vi "LINC Add Packet.vi"(0 "LINC session":refnum<class "LINC.lvclass">, 1 "add header (F)":bool, 2 "type (CMD)":enum16{"CMD", "TLM"}(ring), 5 "item names in":string[](array[string]), 7 "item formats in":T1[](array[typedef]), 9 "hazardous":bool, 11 "e rror in (no error)":errorcluster, 12 "packet name":string, 13 "packet description":string, 14 "ID":i32) -> (4 "dup LINC session":refnum<class "LINC.lvclass">, 15 "error out":errorcluster)   [LabVIEW 2018, in "STEPkgDriver_LINC.lvlib" / "LINC.lvclass"]
uses:
  LINC.lvclass
  STEPkgDriver_LINC.lvlib
  LINC Global Mode.ctl
  LINC Global ID Mode.ctl
  LINC Format Prototype.ctl
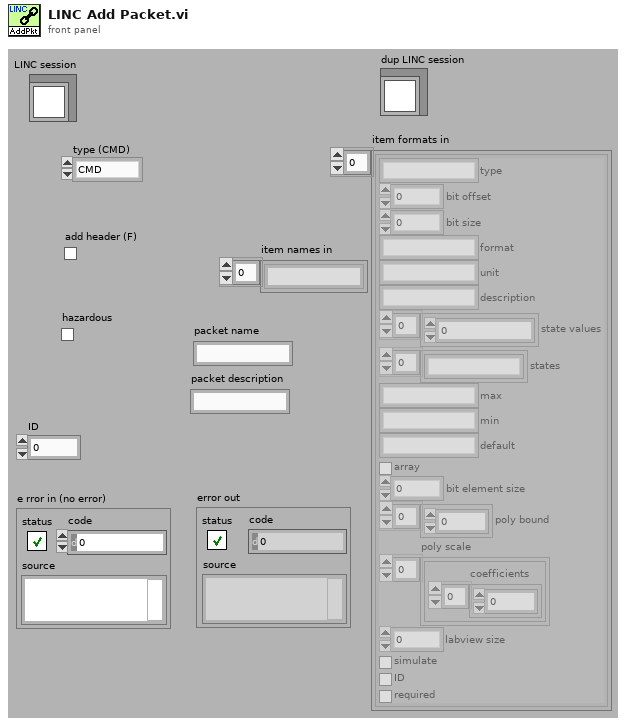
[diagram p1: front panel]
types:
  T1 = typedef "STEPkgDriver_LINC.lvlib/LINC Format Prototype.ctl" = cluster{"type":string, "bit offset":i32, "bit size":i32, "format":string, "unit":string, "description":string, "state values":i64[], "states":string[], "max":string, "min":string, "default":string, "array":bool, "bit element size":i32, "poly bound":dbl[], "poly scale":cluster{"coefficients":dbl[]}[], "labview size":i32, "simulate":bool, "ID":bool, "required":bool}
  T2 = typedef "STEPkgDriver_LINC.lvlib/LINC Global ID Mode.ctl" = enum16{"INIT", "CLEAR", "GET_ID"}
  T3 = typedef "STEPkgDriver_LINC.lvlib/LINC Global Mode.ctl" = enum16{"INIT", "CLEAR", "ADD_PKT_HDR", "ADD_PKT", "GET_PKT_NAMES", "GET_PKT_DESC", "GET_PKT_HDR", "GET_PKT", "SET_PKT", "SET_DATA", "SIM_EN", "SIM_DS"}
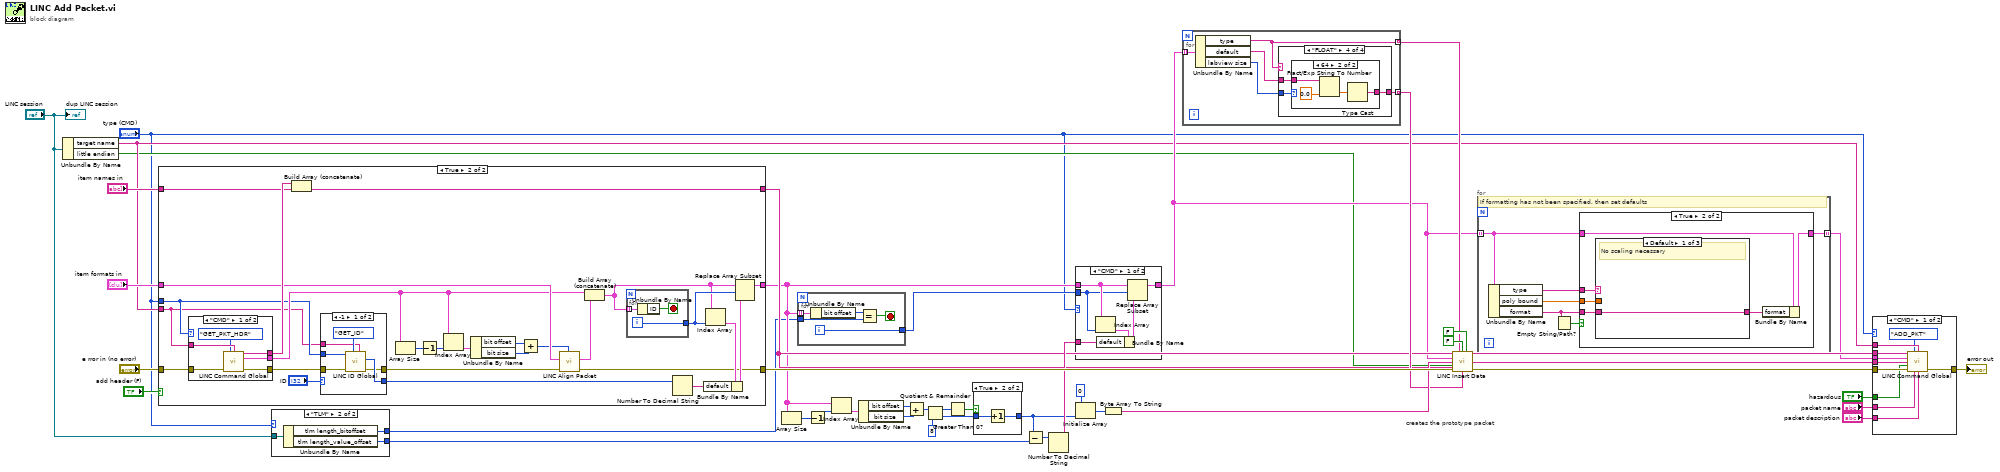
[diagram p0: block diagram]
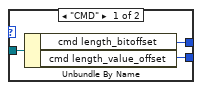
[diagram p4: hidden frame]
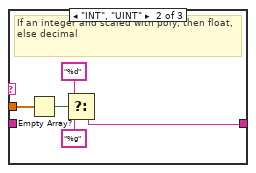
[diagram p6: hidden frame]
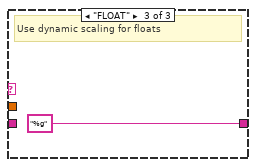
[diagram p7: hidden frame]
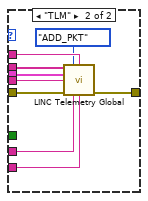
[diagram p8: hidden frame]
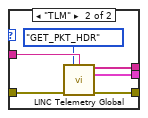
[diagram p11: hidden frame]
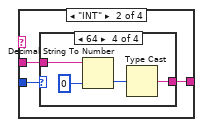
[diagram p13: hidden frame]
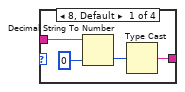
[diagram p14: hidden frame]
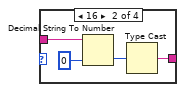
[diagram p15: hidden frame]
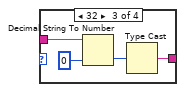
[diagram p16: hidden frame]
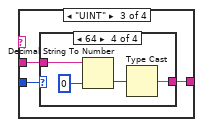
[diagram p17: hidden frame]
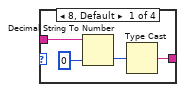
[diagram p18: hidden frame]
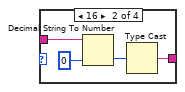
[diagram p19: hidden frame]
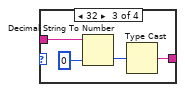
[diagram p20: hidden frame]
diagram:
  # "creates the prototype packet"
  n1 = Unbundle By Name("LINC session") -> ("target name"=w12:string, "little endian"=w7:bool)
  n2 = case shown="True" "add header (F)" {
    tunnel: [w43 w59] -> w40
    tunnel: "e rror in (no error)" -> [w43 w71]
    tunnel: "item names in" -> [w45 w69]
    tunnel: "item formats in" -> [w44 w61]
    tunnel: [w44 w62] -> w16
    tunnel: [w45 w68] -> w20
    tunnel: w12 -> [_ w46]
    tunnel: "type (CMD)" -> [_ w47]
    frame False {
    }
    frame True {
      n3 = case shown="\"CMD\"" w47 {
        tunnel: [w85 w91] -> w50
        tunnel: w71 -> [w84 w90]
        tunnel: [w83 w89] -> w70
        tunnel: [w82 w88] -> w56
        tunnel: w46 -> [w81 w87]
        frame "CMD" {
          n4 = call "LINC Command Global.vi"("mode"=LINC_Global_Mode."GET_PKT_HDR", "target name"=w81, "error in (no error)"=w84) -> ("values out"=w83:string[], "item formats out"=w82:T1[], "error out"=w85:errorcluster)  [unwired: 8 in, 2 out]
        }
        frame "TLM" {
          n5 = call "LINC Telemetry Global.vi"("mode"=LINC_Global_Mode."GET_PKT_HDR", "target name"=w87, "error in (no error)"=w90) -> ("values out"=w89:string[], "item formats out"=w88:T1[], "error out"=w91:errorcluster)  [unwired: 8 in, 2 out]
        }
      }
      n6 = Build Array (concatenate)(w70, w69) -> (w68:string[])
      n7 = case shown="-1" "ID" {
        selector: "ID" -> [_ w79]
        tunnel: [w77 w79] -> w48
        tunnel: [w76 w78] -> w49
        tunnel: w50 -> [w75 w78]
        tunnel: w47 -> [w74 _]
        tunnel: w46 -> [w72 _]
        frame -1 {
          n8 = call "LINC ID Global.vi"("target name"=w72, "mode"=LINC_Global_ID_Mode."GET_ID", "error in (no error)"=w75, "type (CMD)"=w74) -> ("error out"=w76:errorcluster, "ID"=w77:i32)  [unwired: 6 in]
        }
        frame Default {
        }
      }
      n9 = Array Size(array=w56) -> (size(s)=w58:i32)
      n10 = Decrement(x=w58) -> (x-1=w57:i32)
      n11 = Index Array(array=w56, index=w57) -> (element=w55:T1)
      n12 = Unbundle By Name(w55) -> ("bit offset"=w54:i32, "bit size"=w53:i32)
      n13 = Add(x=w54, y=w53) -> (x+y=w52:i32)
      n14 = call "LINC Align Packet.vi"("initial offset"=w52, "error in (no error)"=w49, "item formats in"=w61) -> ("error out"=w59:errorcluster, "item formats out"=w60:T1[])  [unwired: 7 in]
      n15 = Build Array (concatenate)(w56, w60) -> (w63:T1[])
      n16 = for {
        tunnel: w63 -> [w94] mode=indexing
        tunnel: [w92] -> w65
        i -> [w92]
        stop <- w93 stop-if-true
        n17 = Unbundle By Name(w94) -> ("ID"=w93:bool)
      }
      n18 = Number To Decimal String(number=w48) -> (decimal integer string=w67:string)  [unwired: 1 in]
      n19 = Index Array(array=w63, index=w65) -> (element=w66:T1)
      n20 = Bundle By Name(cluster=w66, "default"=w67) -> (w64:T1)
      n21 = Replace Array Subset(array=w63, new element=w64, index=w65) -> (w62:T1[])
    }
  }
  n22 = case shown="\"TLM\"" "type (CMD)" {
    tunnel: [w97 w100] -> w15
    tunnel: [w96 w99] -> w13
    tunnel: "LINC session" -> [w95 w98]
    frame "CMD" {
      n23 = Unbundle By Name(w95) -> ("cmd length_bitoffset"=w97:i32, "cmd length_value_offset"=w96:i32)
    }
    frame "TLM" {
      n24 = Unbundle By Name(w98) -> ("tlm length_bitoffset"=w100:i32, "tlm length_value_offset"=w99:i32)
    }
  }
  n25 = Array Size(array=w16) -> (size(s)=w33:i32)
  n26 = for {
    tunnel: w16 -> [w105] mode=indexing
    tunnel: w15 -> [w103]
    tunnel: [w101] -> w14
    i -> [w101]
    stop <- w102 stop-if-true
    n27 = Unbundle By Name(w105) -> ("bit offset"=w104:i32)
    n28 = Equal?(x=w104, y=w103) -> (x = y?=w102:bool)
  }
  n29 = Decrement(x=w33) -> (x-1=w34:i32)
  n30 = Index Array(array=w16, index=w34) -> (element=w35:T1)
  n31 = Unbundle By Name(w35) -> ("bit offset"=w36:i32, "bit size"=w37:i32)
  n32 = Add(x=w36, y=w37) -> (x+y=w32:i32)
  n33 = Quotient & Remainder(x=w32, y=8) -> (x-y*floor(x/y)=w5:i32, floor(x/y)=w2:i32)
  n34 = Greater Than 0?(x=w5) -> (x > 0?=w4:bool)
  n35 = case shown="True" w4 {
    tunnel: [w106 w107] -> w3
    tunnel: w2 -> [w106 w108]
    frame False {
    }
    frame True {
      n36 = Increment(x=w108) -> (x+1=w107:i32)
    }
  }
  n37 = Subtract(x=w3, y=w13) -> (x-y=w30:i32)
  n38 = Number To Decimal String(number=w30) -> (decimal integer string=w29:string)  [unwired: 1 in]
  n39 = case shown="\"CMD\"" "type (CMD)" {
    tunnel: w29 -> [w112 _]
    tunnel: [w111 w115] -> w18
    tunnel: w16 -> [w110 w115]
    tunnel: w14 -> [w109 _]
    frame "CMD" {
      n40 = Index Array(array=w110, index=w109) -> (element=w114:T1)
      n41 = Bundle By Name(cluster=w114, "default"=w112) -> (w113:T1)
      n42 = Replace Array Subset(array=w110, new element=w113, index=w109) -> (w111:T1[])
    }
    frame "TLM" {
    }
  }
  n43 = Initialize Array(u8 0, w3) -> (w27:u8[])
  n44 = Byte Array To String(unsigned byte array=w27) -> (string=w26:string)
  n45 = for {
    tunnel: w18 -> [w120] mode=indexing
    tunnel: [w119] -> w25 mode=indexing
    tunnel: [w117] -> w24 mode=indexing
    n46 = Unbundle By Name(w120) -> ("type"=w119:string, "default"=w118:string, "labview size"=w116:i32)
    n47 = case shown="\"FLOAT\"" w119 {
      tunnel: w118 -> [w121 w124 w143 w162]
      tunnel: [w121 w123 w142 w161] -> w117
      tunnel: w116 -> [_ w122 w141 w160]
      frame Default {
      }
      frame "INT" {
        n48 = case shown="64" w122 {
          tunnel: w124 -> [w128 w132 w136 w140]
          tunnel: [w125 w129 w133 w137] -> w123
          frame 8, Default {
            n49 = Decimal String To Number(string=w128, default (0L)=i8 0) -> (number=w126:i8)  [unwired: 1 in, 1 out]
            n50 = Type Cast(x=w126) -> (*(type *) &x=w125:string)  [unwired: 1 in]
          }
          frame 16 {
            n51 = Decimal String To Number(string=w132, default (0L)=i16 0) -> (number=w130:i16)  [unwired: 1 in, 1 out]
            n52 = Type Cast(x=w130) -> (*(type *) &x=w129:string)  [unwired: 1 in]
          }
          frame 32 {
            n53 = Decimal String To Number(string=w136, default (0L)=0) -> (number=w134:i32)  [unwired: 1 in, 1 out]
            n54 = Type Cast(x=w134) -> (*(type *) &x=w133:string)  [unwired: 1 in]
          }
          frame 64 {
            n55 = Decimal String To Number(string=w140, default (0L)=i64 0) -> (number=w138:i64)  [unwired: 1 in, 1 out]
            n56 = Type Cast(x=w138) -> (*(type *) &x=w137:string)  [unwired: 1 in]
          }
        }
      }
      frame "UINT" {
        n57 = case shown="64" w141 {
          tunnel: w143 -> [w147 w151 w155 w159]
          tunnel: [w144 w148 w152 w156] -> w142
          frame 8, Default {
            n58 = Decimal String To Number(string=w147, default (0L)=u8 0) -> (number=w145:u8)  [unwired: 1 in, 1 out]
            n59 = Type Cast(x=w145) -> (*(type *) &x=w144:string)  [unwired: 1 in]
          }
          frame 16 {
            n60 = Decimal String To Number(string=w151, default (0L)=u16 0) -> (number=w149:u16)  [unwired: 1 in, 1 out]
            n61 = Type Cast(x=w149) -> (*(type *) &x=w148:string)  [unwired: 1 in]
          }
          frame 32 {
            n62 = Decimal String To Number(string=w155, default (0L)=u32 0) -> (number=w153:u32)  [unwired: 1 in, 1 out]
            n63 = Type Cast(x=w153) -> (*(type *) &x=w152:string)  [unwired: 1 in]
          }
          frame 64 {
            n64 = Decimal String To Number(string=w159, default (0L)=u64 0) -> (number=w157:u64)  [unwired: 1 in, 1 out]
            n65 = Type Cast(x=w157) -> (*(type *) &x=w156:string)  [unwired: 1 in]
          }
        }
      }
      frame "FLOAT" {
        n66 = case shown="64" w160 {
          tunnel: w162 -> [w166 w170]
          tunnel: [w163 w167] -> w161
          frame 32, Default {
            n67 = Fract/Exp String To Number(string=w166, default (0 dbl)=sgl 0.0) -> (number=w164:sgl)  [unwired: 2 in, 1 out]
            n68 = Type Cast(x=w164) -> (*(type *) &x=w163:string)  [unwired: 1 in]
          }
          frame 64 {
            n69 = Fract/Exp String To Number(string=w170, default (0 dbl)=0.0) -> (number=w168:dbl)  [unwired: 2 in, 1 out]
            n70 = Type Cast(x=w168) -> (*(type *) &x=w167:string)  [unwired: 1 in]
          }
        }
      }
    }
  }
  n71 = call "LINC Insert Data.vi"("item names"=w20, "member types"=w25, "scale"=FALSE, "simulate"=FALSE, "item formats"=w18, "data in"=w26, "little endian"=w7, "error in (no error)"=w40, "member names"=w20, "member data"=w24) -> ("data out"=w19:string, "error out"=w22:errorcluster)  [unwired: 4 in]
  n72 = for {
    tunnel: w18 -> [w175] mode=indexing
    tunnel: [w174] -> w17 mode=indexing
    # "If formatting has not been specified, then set defaults"
    n73 = Unbundle By Name(w175) -> ("type"=w173:string, "poly bound"=w171:dbl[], "format"=w172:string)
    n74 = Empty String/Path?(string/path=w172) -> (empty?=w176:bool)
    n75 = case shown="True" w176 {
      tunnel: w175 -> [w177 w182]
      tunnel: [w177 w181] -> w174
      tunnel: w173 -> [_ w183]
      tunnel: w172 -> [_ w179]
      tunnel: w171 -> [_ w178]
      frame False {
      }
      frame True {
        n76 = case shown="Default" w183 {
          tunnel: [w184 w187 "%g" ("y")] -> w180
          tunnel: w179 -> [w184 _ _]
          tunnel: w178 -> [_ w189 _]
          frame Default {
            # "No scaling necessary"
          }
          frame "INT", "UINT" {
            # "If an integer and scaled with poly, then float, else decimal"
            n77 = Empty Array?(array=w189) -> (empty?=w188:bool)
            n78 = Select(t="%d" ("y"), s=w188, f="%g" ("y")) -> (s? t:f=w187:string)
          }
          frame "FLOAT" {
            # "Use dynamic scaling for floats"
          }
        }
        n79 = Bundle By Name(cluster=w182, "format"=w180) -> (w181:T1)
      }
    }
  }
  n80 = case shown="\"CMD\"" "type (CMD)" {
    tunnel: [w200 w209] -> w21
    tunnel: w22 -> [w199 w208]
    tunnel: w12 -> [w198 w207]
    tunnel: w20 -> [w196 w205]
    tunnel: w17 -> [w195 w204]
    tunnel: w19 -> [w194 w203]
    tunnel: "packet name" -> [w193 w202]
    tunnel: "packet description" -> [w192 w201]
    tunnel: "hazardous" -> [w191 _]
    frame "CMD" {
      n81 = call "LINC Command Global.vi"("item names in"=w196, "mode"=LINC_Global_Mode."ADD_PKT", "target name"=w198, "item formats in"=w195, "data in"=w194, "hazardous in"=w191, "error in (no error)"=w199, "packet name"=w193, "packet description"=w192) -> ("error out"=w200:errorcluster)  [unwired: 2 in, 4 out]
    }
    frame "TLM" {
      n82 = call "LINC Telemetry Global.vi"("item names in"=w205, "mode"=LINC_Global_Mode."ADD_PKT", "target name"=w207, "item formats in"=w204, "data in"=w203, "error in (no error)"=w208, "packet name"=w202, "packet description"=w201) -> ("error out"=w209:errorcluster)  [unwired: 3 in, 4 out]
    }
  }
  "error out" <- w21
  "dup LINC session" <- "LINC session"
